vi "Rechteck-Koordinaten ordnen.vi"(7 "Rechteck-Koordinaten":T1) -> (3 "Koordinaten geordnet":T1)   [LabVIEW 2020, in "Anlagenuebersicht.lvlib" / "VisBx Anzeige.lvlib"]
uses:
  VisBx Anzeige.lvlib
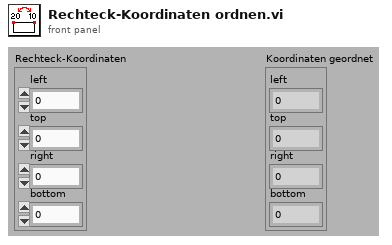
[diagram p1: front panel]
types:
  T1 = cluster{"left":i16, "top":i16, "right":i16, "bottom":i16}
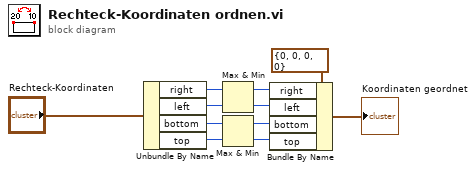
[diagram p0: block diagram]
diagram:
  n1 = Unbundle By Name("Rechteck-Koordinaten") -> ("right"=w6:i16, "left"=w7:i16, "bottom"=w8:i16, "top"=w9:i16)
  n2 = Max & Min(x=w6, y=w7) -> (max(x,y)=w4:i16, min(x,y)=w5:i16)
  n3 = Max & Min(x=w8, y=w9) -> (max(x,y)=w10:i16, min(x,y)=w11:i16)
  n4 = Bundle By Name(cluster=T1 {"left"=0, "top"=0, "right"=0, "bottom"=0} ("rect"), "right"=w4, "left"=w5, "bottom"=w10, "top"=w11) -> (→"Koordinaten geordnet":T1)
